vi "Read Output.vi"(0 "VISA resource name":refnum<visa-resource-name>, 5 "Channel Select":enum16{"Channel 1", "Channel 2", "Channel 3"}(ring), 7 "Measurement Function (0:Voltage)":u16(ring) items=["Voltage", "Current", "Power"], 11 "error in (no error)":errorcluster) -> (4 "VISA resource name out":refnum<visa-resource-name>, 6 "Measurement":string, 15 "error out":errorcluster)   [LabVIEW 2018, in "Keithley KE22xx Series.lvlib"]
doc: "Read the response from the instrument as per the selected parameter."
uses:
  Keithley KE22xx Series.lvlib
panel:
  # "© 2012 Keithley Instruments, Inc. ALL RIGHTS RESERVED"
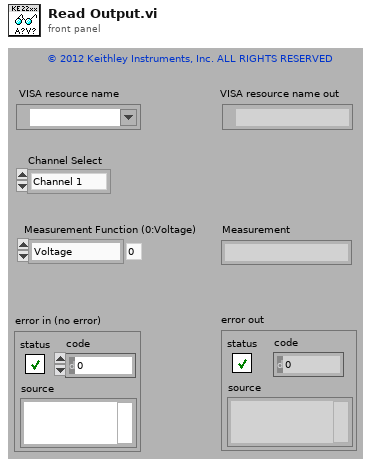
[diagram p1: front panel]
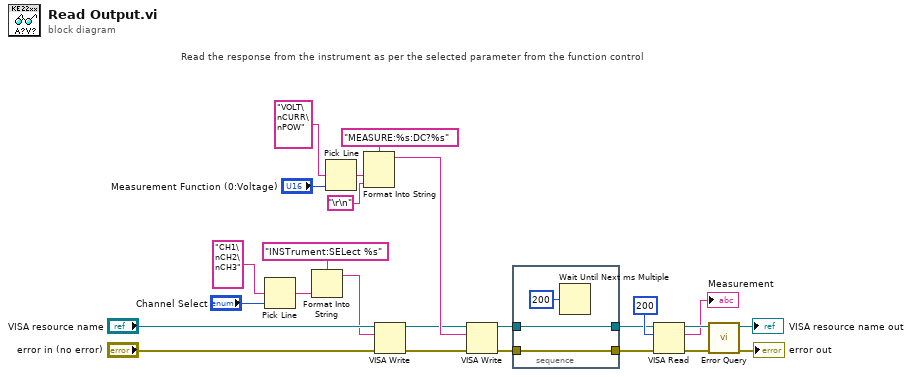
[diagram p0: block diagram]
diagram:
  # "Read the response from the instrument as per the selected parameter from the function control"
  n1 = Pick Line(multi-line string="CH1\nCH2\nCH3", line index="Channel Select") -> (output string=w8:string)  [unwired: 1 in]
  n2 = Format Into String(format string="INSTrument:SELect %s", w8) -> (resulting string=w2:string)  [unwired: 2 in, 1 out]
  n3 = Pick Line(multi-line string="VOLT\nCURR\nPOW" ("write buffer"), line index="Measurement Function (0:Voltage)") -> (output string=w13:string)  [unwired: 1 out]
  n4 = Format Into String(format string="MEASURE:%s:DC?%s", w13, "\r\n") -> (resulting string=w10:string)  [unwired: 2 in, 1 out]
  n5 = VISA Write(VISA resource name="VISA resource name", write buffer=w2, error in (no error)="error in (no error)") -> (VISA resource name out=w3:refnum<visa-resource-name>, error out=w4:errorcluster)  [unwired: 1 out]
  n6 = VISA Write(VISA resource name=w3, write buffer=w10, error in (no error)=w4) -> (VISA resource name out=w20:refnum<visa-resource-name>, error out=w18:errorcluster)  [unwired: 1 out]
  n7 = stacked-sequence {
    tunnel: [w28] -> w19
    tunnel: w20 -> [w28]
    tunnel: w18 -> [w27]
    tunnel: [w27] -> w17
    frame #0 {
      n8 = Wait Until Next ms Multiple(millisecond multiple=u32 200 ("Programmable Delay in ms")) -> ()  [unwired: 1 out]
    }
  }
  n9 = VISA Read(VISA resource name=w19, byte count=u32 200, error in (no error)=w17) -> (VISA resource name out=w23:refnum<visa-resource-name>, read buffer=→"Measurement":string, error out=w22:errorcluster)  [unwired: 1 out]
  n10 = call "Error Query.vi"("error in (no error)"=w22, "VISA resource name"=w23) -> ("error out"=→"error out":errorcluster, "VISA resource name out"=→"VISA resource name out":refnum<visa-resource-name>)  [unwired: 6 in, 2 out]
